vi "Write portNumber.vi"(8 "error in (no error)":errorcluster, 10 "portNumber":u8 max=1, 11 "WriteAnalog in":refnum<class "WriteAnalog.lvclass">) -> (0 "error out":errorcluster, 3 "WriteAnalog out":refnum<class "WriteAnalog.lvclass">)   [LabVIEW 2013, in "MaterialCharacterization.lvlib" / "WriteAnalog.lvclass"]
uses:
  WriteAnalog.lvclass
  WriteAnalog.lvclass/WriteAnalog.ctl
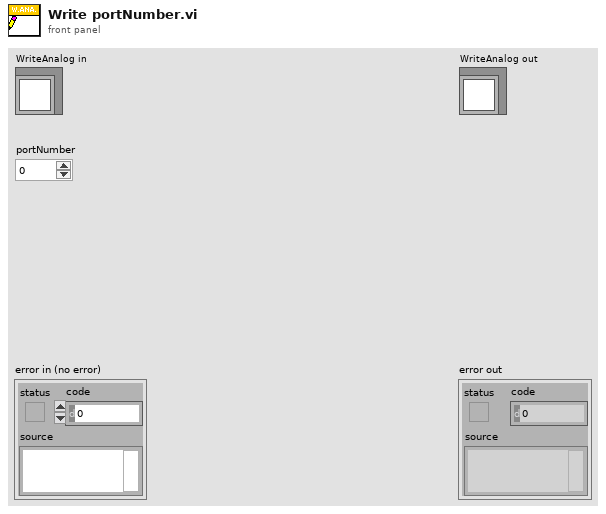
[diagram p1: front panel]
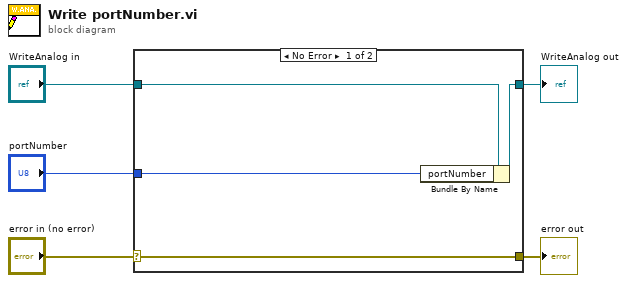
[diagram p0: block diagram]
diagram:
  n1 = case shown="No Error" "error in (no error)" {
    selector: "error in (no error)" -> [w9 w10]
    tunnel: [w9 w10] -> w4
    tunnel: [w7 w11] -> w2
    tunnel: "WriteAnalog in" -> [w8 w11]
    tunnel: "portNumber" -> [w6 _]
    frame No Error {
      n2 = Bundle By Name(cluster=w8, "portNumber"=w6) -> (w7:refnum<class "WriteAnalog.lvclass">)
    }
    frame Error {
    }
  }
  "error out" <- w4
  "WriteAnalog out" <- w2
